vi "BackwardsPropLR.vi"(6 "Target":dbl[](array[numeric]), 7 "Learning Rate":dbl, 9 "Input":dbl[](array[numeric]), 10 "Y vectors":cluster{dbl[]}[](array[cluster]), 11 "Weights":cluster{"A - B":T1}[](array[cluster])) -> (2 "Array 2":cluster{"Outer Product":T1}[](array[cluster]), 3 "Array":cluster{"A - B":T1}[](array[cluster]))   [LabVIEW 2016]
uses:
  <vilib>/Analysis/Matrix/Datatypes/RealMatrix.ctl
  <vilib>/Analysis/baseanly.llb/Vector x A.vi
  <vilib>/Analysis/baseanly.llb/Real Outer Product.vi
  <vilib>/Analysis/Matrix/Numeric/Multiply/Multiply - RM,R.vi
  <vilib>/Analysis/Matrix/Numeric/Subtract/Subtract - RM,RM.vi
  <vilib>/Analysis/NI_AALBase.lvlib
  <vilib>/Analysis/Matrix/NI_Matrix.lvlib
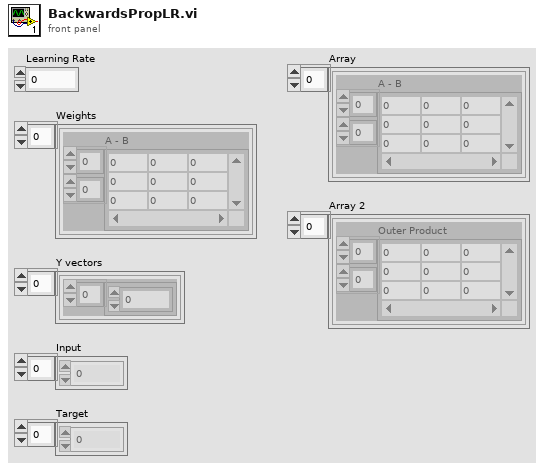
[diagram p1: front panel]
types:
  T1 = typedef "NI_Matrix.lvlib/RealMatrix.ctl" = dbl[][]
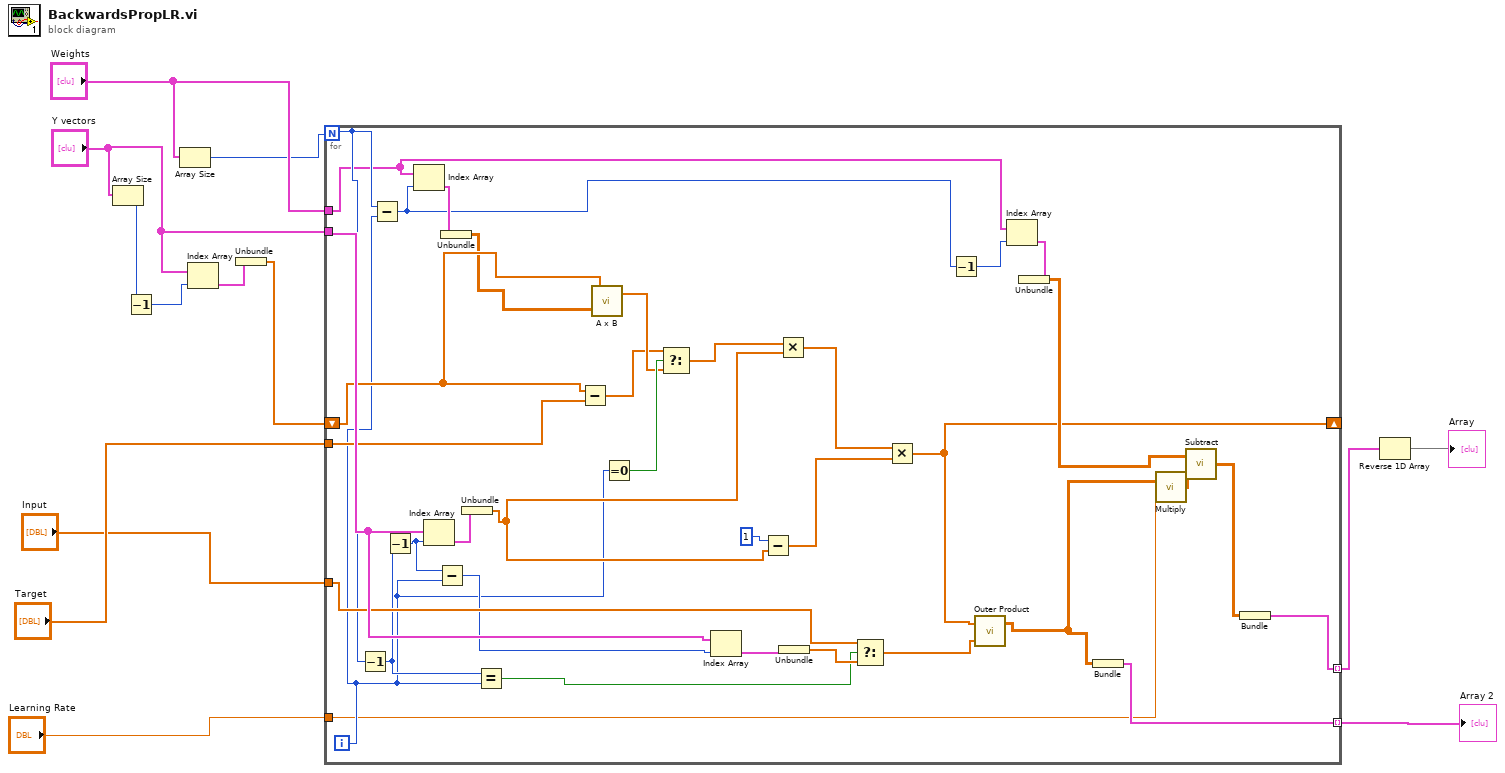
[diagram p0: block diagram]
diagram:
  n1 = Array Size(array="Y vectors") -> (size(s)=w11:i32)
  n2 = Decrement(x=w11) -> (x-1=w10:i32)
  n3 = Array Size(array="Weights") -> (size(s)=w7:i32)
  n4 = Index Array(array="Y vectors", index=w10) -> (element=w12:cluster{dbl[]})
  n5 = Unbundle(w12) -> (w6:dbl[])
  n6 = for {
    N: w7 -> [w29]
    tunnel: "Weights" -> [w25]
    tunnel: "Y vectors" -> [w49]
    tunnel: "Input" -> [w48]
    shift-right: [w20] -> _
    shift-left: w6 -> [w37]
    tunnel: "Target" -> [w36]
    tunnel: [w16] -> w2 mode=indexing
    tunnel: [w15] -> w1 mode=indexing
    tunnel: "Learning Rate" -> [w14]
    i -> [w28]
    n7 = Decrement(x=w29) -> (x-1=w30:i32)
    n8 = Subtract(x=w29, y=w28) -> (x-y=w27:i32)
    n9 = Decrement(x=w30) -> (x-1=w39:i32)
    n10 = Index Array(array=w25, index=w27) -> (element=w47:cluster{"A - B":T1})
    n11 = Index Array(array=w49, index=w39) -> (element=w44:cluster{dbl[]})
    n12 = Subtract(x=w39, y=w28) -> (x-y=w38:i32)
    n13 = Unbundle(w47) -> ("A - B"=w31:T1)
    n14 = Unbundle(w44) -> (w43:dbl[])
    n15 = Equal?(x=w30, y=w28) -> (x = y?=w40:bool)
    n16 = Subtract(x=w37, y=w36) -> (x-y=w33:dbl[])
    n17 = call-poly <vilib>:"A x B.vi"("Matrix A"=w31, "Vector V'"=w37) -> ("V' x A"=w34:dbl[])  [unwired: 1 out]
    n18 = Equal To 0?(x=w28) -> (x = 0?=w35:bool)
    n19 = Select(t=w33, s=w35, f=w34) -> (s? t:f=w32:dbl[])
    n20 = Index Array(array=w49, index=w38) -> (element=w46:cluster{dbl[]})
    n21 = Subtract(x=1, y=w43) -> (x-y=w42:dbl[])
    n22 = Multiply(x=w32, y=w43) -> (x*y=w45:dbl[])
    n23 = Unbundle(w46) -> (w41:dbl[])
    n24 = Select(t=w48, s=w40, f=w41) -> (s? t:f=w21:dbl[])
    n25 = Multiply(x=w45, y=w42) -> (x*y=w20:dbl[])
    n26 = Decrement(x=w27) -> (x-1=w26:i32)
    n27 = call-poly <vilib>:"Outer Product.vi"("Y Vector"=w21, "X Vector"=w20) -> ("Outer Product"=w19:T1)  [unwired: 1 out]
    n28 = Index Array(array=w25, index=w26) -> (element=w24:cluster{"A - B":T1})
    n29 = Unbundle(w24) -> ("A - B"=w22:T1)
    n30 = Bundle("Outer Product"=w19) -> (w15:cluster{"Outer Product":T1})  [unwired: 1 in]
    n31 = call-poly <vilib>:"Multiply.vi"("Real Scalar c"=w14, "Real Matrix A"=w19) -> ("A * c"=w17:T1)
    n32 = call-poly <vilib>:"Subtract.vi"("Real Matrix B"=w17, "Real Matrix A"=w22) -> ("A - B"=w23:T1)
    n33 = Bundle("A - B"=w23) -> (w16:cluster{"A - B":T1})  [unwired: 1 in]
  }
  "Array 2" <- w1
  n34 = Reverse 1D Array(array=w2) -> (reversed array=→"Array":cluster{"A - B":T1}[])
